vi "Time Estimate.vi"(8 "error in (no error)":errorcluster, 9 "expmode":i32, 10 "scantype":T1(ring), 11 "Double Scanner.lvclass":refnum<class "Double Scanner.lvclass">) -> (0 "error out":errorcluster, 1 "Time Estimate":string, 2 "time":dbl[unit], 3 "Double Scanner.lvclass out":refnum<class "Double Scanner.lvclass">)   [LabVIEW 2017, in "Double Scanner.lvclass"]
doc: "(Dynamic) Return an estimate of the time remaining to scan over this Scanner's preconfigured Range."
uses:
  Double Scanner.lvclass
  Scanner/Scanner.lvclass
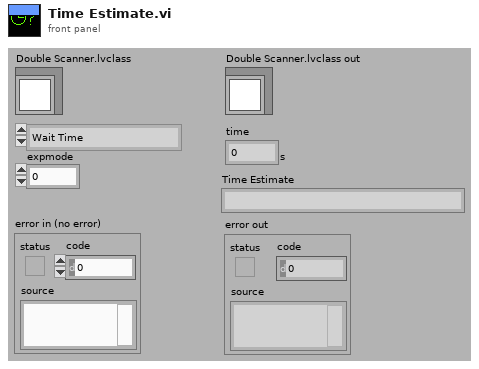
[diagram p1: front panel]
types:
  T1 = enum16{"Wait Time", "Pulse Width", "Wavelength", "Magnetic Field", "rf Scan"}
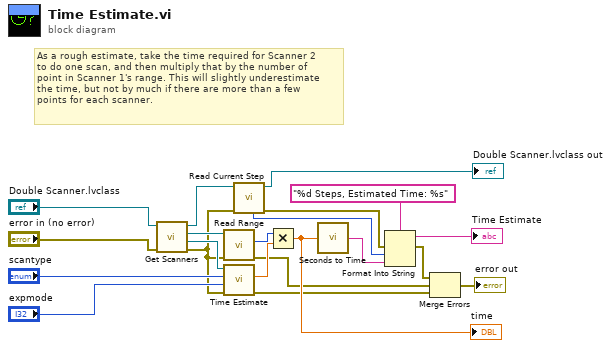
[diagram p0: block diagram]
diagram:
  # "As a rough estimate, take the time required for Scanner 2\nto do one scan, and then multiply that by the number of\npoint in Scanner 1's range. This will slightly underestimate\nthe time, but not by much if there are more than a few\npoints for each scanner."
  n1 = call-dynamic "Get Scanners.vi"("error in (no error)"="error in (no error)", "Double Scanner in"="Double Scanner.lvclass") -> ("error out"=w10:errorcluster, "Scanner 2 out"=w21:refnum<class "Scanner.lvclass">, "Scanner 1 out"=w20:refnum<class "Scanner.lvclass">, "Double Scanner out"=w11:refnum<class "Double Scanner.lvclass">)  [unwired: 6 in]
  n2 = call-dynamic "Read Range.vi"("error in (no error)"=w10, "Scanner.lvclass in"=w20) -> ("error out"=w4:errorcluster, "# Points"=w19:u32)  [unwired: 4 in, 4 out]
  n3 = call-dynamic "Time Estimate.vi"("error in (no error)"=w10, "expmode"="expmode", "scantype"="scantype", "Scanner.lvclass"=w21) -> ("error out"=w3:errorcluster, "time"=w18:dbl[unit])  [unwired: 4 in, 2 out]
  n4 = call-dynamic "Read Current Step.vi"("error in (no error)"=w10, "Double Scanner in"=w11) -> ("error out"=w5:errorcluster, "Double Scanner out"=→"Double Scanner.lvclass out":refnum<class "Double Scanner.lvclass">, "Total steps"=w7:i32)  [unwired: 5 in, 2 out]
  n5 = Multiply(x=w19, y=w18) -> (x*y=w17:dbl[unit])
  "time" <- w17
  n6 = call "Seconds to Time.vi"("Seconds"=w17) -> ("Time"=w8:string)
  n7 = Format Into String(format string="%d Steps, Estimated Time: %s", error in=w5, w7, w8) -> (resulting string=→"Time Estimate":string, error out=w2:errorcluster)  [unwired: 1 in]
  n8 = Merge Errors(w2, w4, w3) -> (→"error out":errorcluster)
